vi "Matrix-Pose.vi"(8 "error in":errorcluster, 11 "T":T1=[[0.016284994521607307, 0.9998576764567041, 0.0044074691186384496, -12.095922523672678], [0.9998670931969393, -0.01628143110047913, -0.0008431744914288715, -1019.3924117975101], [-0.0007712945830650122, 0.004420614427981981, -0.999989931585686, 240.25900755427352], [0.0, 0.0, 0.0, 1.0]] format="%.3f") -> (0 "error out":errorcluster, 3 "pose":dbl[][](array[numeric]))   [LabVIEW 2013]
uses:
  <vilib>/Analysis/Matrix/Datatypes/RealMatrix.ctl
  <vilib>/Analysis/Matrix/NI_Matrix.lvlib
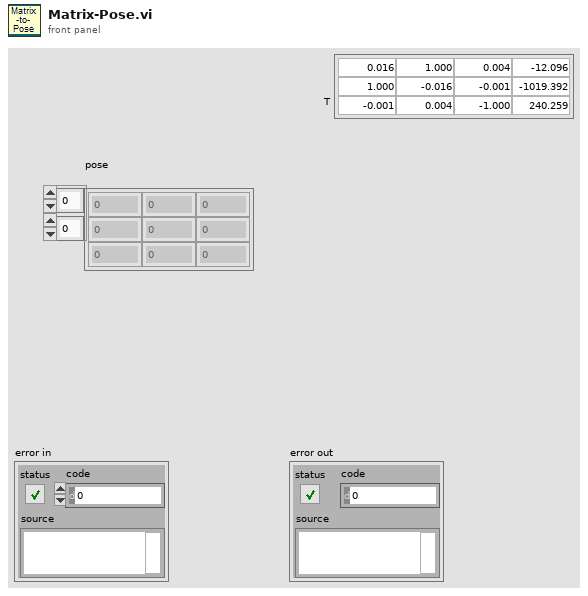
[diagram p1: front panel]
types:
  T1 = typedef "NI_Matrix.lvlib/RealMatrix.ctl" = dbl[][]
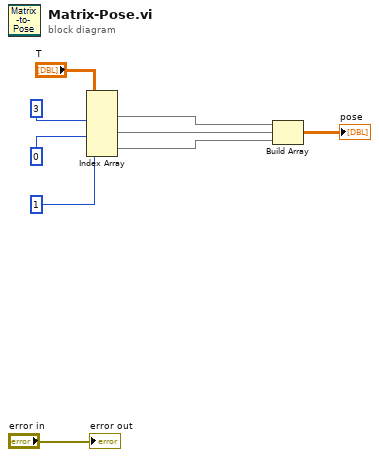
[diagram p0: block diagram]
diagram:
  n1 = Index Array(array="T", index (col) #1=3 ("index (row)"), index (col) #2=0 ("index (row)"), index (col) #3=1 ("index (row)")) -> (element #1=w3:dbl[], element #2=w2:dbl[], element #3=w1:dbl[])  [unwired: 3 in]
  n2 = Build Array(w3, w2, w1) -> (→"pose":dbl[][])
  "error out" <- "error in"
